vi "Memory.Pointer.New Offset Pointer.vi"(8 "error in (no error)":errorcluster, 10 "offset":i64 format="%d bytes", 11 "Pointer in":refnum<class "Memory.Pointer.lvclass">) -> (0 "error out":errorcluster, 2 "offset Pointer":refnum<class "Memory.Pointer.lvclass">, 3 "Pointer out":refnum<class "Memory.Pointer.lvclass">)   [LabVIEW 2016, in "LabVIEW Memory Manager.lvlib" / "Memory.Pointer.lvclass"]
uses:
  Memory.Pointer.lvclass
  Memory.Pointer.lvclass/Memory.Pointer.ctl
  Accessors/Memory.Pointer.Set Address.vi
  Memory.Pointer.Offset to Address.vi
  Accessors/Memory.Pointer.Get Address.vi
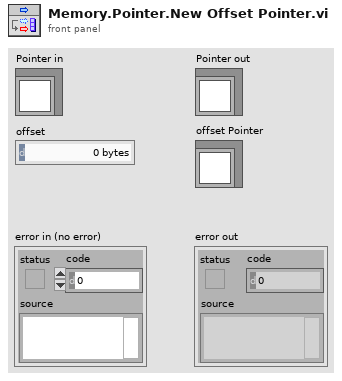
[diagram p1: front panel]
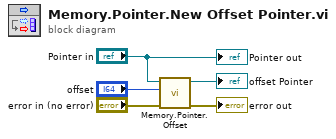
[diagram p0: block diagram]
diagram:
  n1 = call "Memory.Pointer.Offset.vi"("error in (no error)"="error in (no error)", "offset"="offset", "Pointer in"="Pointer in") -> ("error out"=→"error out":errorcluster, "Pointer out"=→"offset Pointer":refnum<class "Memory.Pointer.lvclass">)  [unwired: 7 in]
  "Pointer out" <- "Pointer in"
